vi "SubVI_ExecuteAuto_Auto.vi"(8 "error in (no error)":errorcluster) -> (0 "error out":errorcluster, 1 "String Array":string[](array[string]))   [LabVIEW 2017]
uses:
  <vilib>/Rock Robotics/Network Tables/NT Read String Array.vi
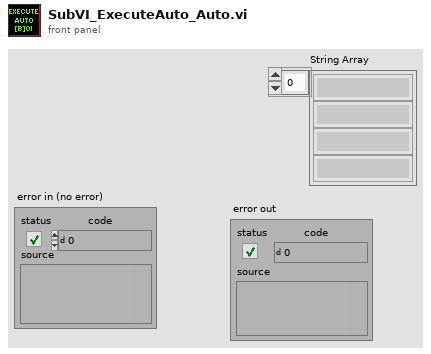
[diagram p1: front panel]
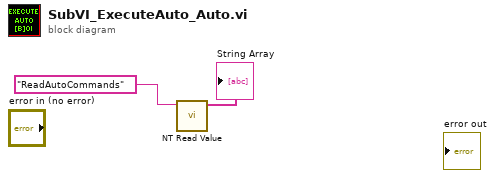
[diagram p0: block diagram]
diagram:
  n1 = call-poly <vilib>:"NT Read Value.vi"("Name"="ReadAutoCommands") -> ("String Array"=→"String Array":string[])  [unwired: 9 in, 1 out]
